vi "PicowattAVS47_Splitt_Cluster.vi"(0 "Picowatt AVS47/TS530 Cluster":T3 {"AVS Excitation" items=["no Exc", "3uV", "10uV", "30uV", "100uV", "300uV", "1mV", "3mV"]}) -> (1 "AVS47 Control Cluster":T1 {"AVS Excitation" items=["no Exc.", "3uV", "10uV", "30uV", "100uV", "300uV", "1mV", "3mV"]}, 2 "AVS47 Status Cluster":T2)   [LabVIEW 2019]
uses:
  PicowattAVS47/PicowattAVS47-Cluster.ctl
  PicowattAVS47/AVS47-Status-Cluster.ctl
  PicowattAVS47/AVS-Control-Cluster.ctl
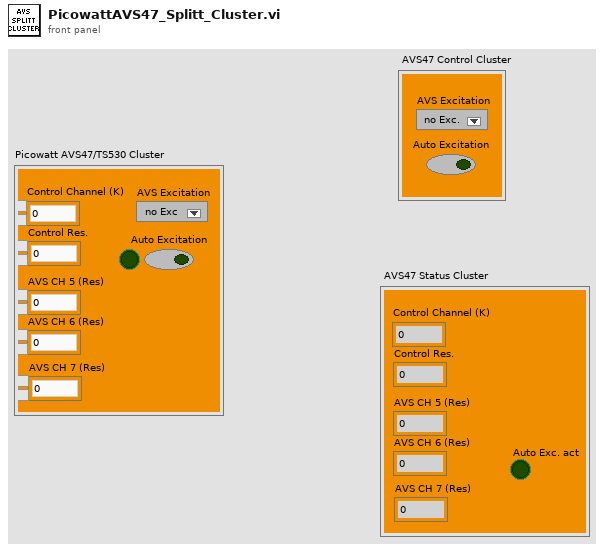
[diagram p1: front panel]
types:
  T1 = typedef "AVS-Control-Cluster.ctl" = cluster{"AVS Excitation":i16, "Auto Excitation":bool}
  T2 = typedef "AVS47-Status-Cluster.ctl" = cluster{"Control Channel (K)":dbl, "AVS CH 5 (Res)":dbl, "AVS CH 6 (Res) ":dbl, "AVS CH 7 (Res) ":dbl, "Control Res.":dbl, "Auto Exc. act":bool}
  T3 = typedef "PicowattAVS47-Cluster.ctl" = cluster{"Control Channel (K)":dbl, "AVS CH 5 (Res)":dbl, "AVS CH 6 (Res) ":dbl, "AVS CH 7 (Res) ":dbl, "Control Res.":dbl, "Auto Excitation":bool, "Auto activatet":bool, "AVS Excitation":i16}
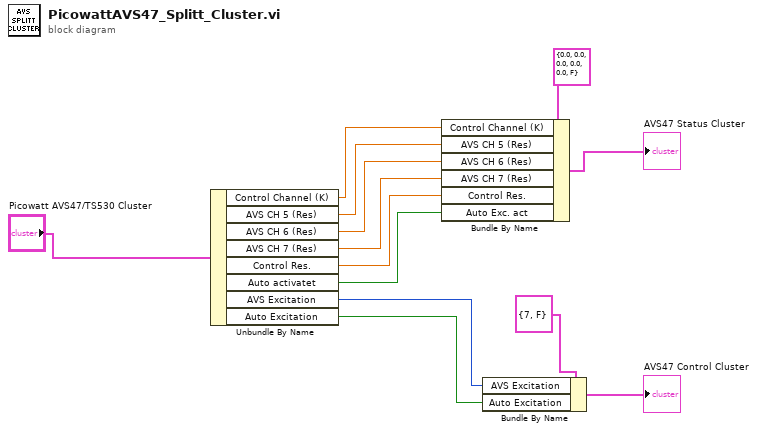
[diagram p0: block diagram]
diagram:
  n1 = Unbundle By Name("Picowatt AVS47/TS530 Cluster") -> ("Control Channel (K)"=w8:dbl, "AVS CH 5 (Res)"=w7:dbl, "AVS CH 6 (Res)"=w6:dbl, "AVS CH 7 (Res)"=w5:dbl, "Control Res."=w4:dbl, "Auto activatet"=w3:bool, "AVS Excitation"=w2:i16, "Auto Excitation"=w1:bool)
  n2 = Bundle By Name(cluster=T2 {"Control Channel (K)"=0.0, "AVS CH 5 (Res)"=0.0, "AVS CH 6 (Res) "=0.0, "AVS CH 7 (Res) "=0.0, "Control Res."=0.0, "Auto Exc. act"=FALSE} ("AVS47 Status Cluster"), "Control Channel (K)"=w8, "AVS CH 5 (Res)"=w7, "AVS CH 6 (Res)"=w6, "AVS CH 7 (Res)"=w5, "Control Res."=w4, "Auto Exc. act"=w3) -> (→"AVS47 Status Cluster":T2)
  n3 = Bundle By Name(cluster=T1 {"AVS Excitation"=7, "Auto Excitation"=FALSE} ("AVS47 Control Cluster"), "AVS Excitation"=w2, "Auto Excitation"=w1) -> (→"AVS47 Control Cluster":T1)
